vi "Max Velocity Reading.vi"() -> ()   [LabVIEW 2018]
uses:
  <vilib>/Rock Robotics/WPI/ThirdParty/Phoenix-LabVIEW/Motor Controller/Controls/CTRE_Phoenix_MotorControl_StatusFrameEnhanced.ctl
  2019_Robot_Code/Subsystems/Drive/driveShifterEnum.ctl
  <vilib>/Rock Robotics/WPI/ThirdParty/Phoenix-LabVIEW/Motor Controller/Get/CTRE_Phoenix_MotorController_GetQuadratureData.vi
panel:
  out "left Velocity (Raw Data)":i32
  out "right Velocity (Raw Data)":i32
  out "Left Max Velocity":dbl
  out "Right Max Velocity":dbl
  out "Left Max Velocity":dbl(graph)
  out "Right Max Velocity":dbl(graph)
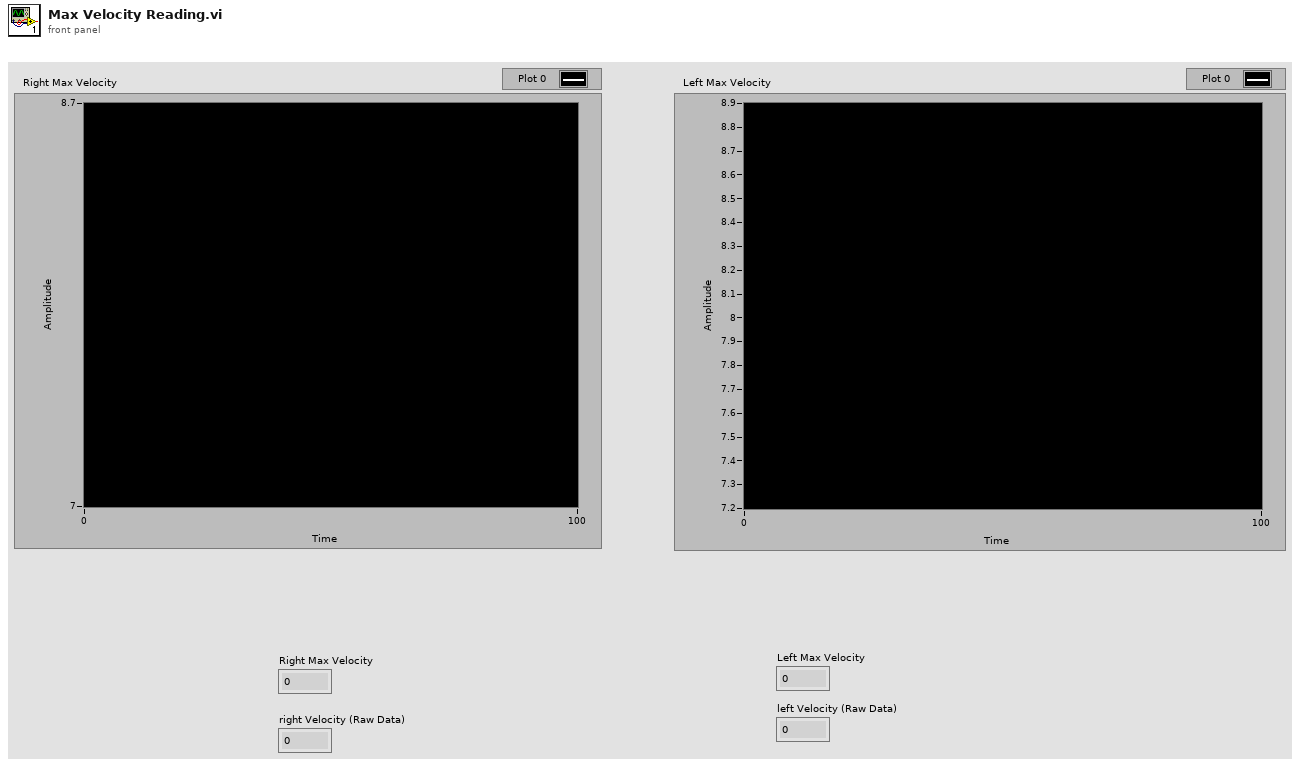
[diagram p1: front panel]
types:
  T1 = typedef "CTRE_Phoenix_MotorControl_StatusFrameEnhanced.ctl" = u16
  T2 = typedef "WPI_MotorControlDeviceRef.ctl" = cluster{"DeviceStatus":errorcluster, "Type":T3, "PWM":cluster{"PWM Channel":T4, "DeadBand":T5}, "CAN":cluster{"Device Number":u8, "SetOutput VI Ref":variant, "GetOutput VI Ref":variant, "Enable VI Ref":variant, "Disable VI Ref":variant, "Data":variant}, "Invert":bool, "DIO PWM":cluster{"PWM \"Enable\" Channel":T4, "DIOChannel":T6, "PWM Rate":dbl}}
  T3 = typedef "WPI_MotorControlType.ctl" = enum16{"PWM", "CAN", "DIO PWM"}
  T4 = typedef "FPGA_DIOPWMChannel.ctl" = enum8{"PWM 0", "PWM 1", "PWM 2", "PWM 3", "PWM 4", "PWM 5", "PWM 6", "PWM 7", "PWM 8", "PWM 9", "PWM MXP 0", "PWM MXP 1", "PWM MXP 2", "PWM MXP 3", "PWM MXP 4", "PWM MXP 5", "PWM MXP 6", "PWM MXP 7", "PWM MXP 8", "PWM MXP 9", "Invalid"}
  T5 = typedef "WPI_PWMDeadband.ctl" = cluster{"Name":string, "maxPositivePwm":i32, "minPositivePwm":i32, "centerPwm":i32, "maxNegativePwm":i32, "minNegativePwm":i32, "angularRange":u16}
  T6 = typedef "FPGA_DIOChannel.ctl" = enum8{"DIO 0", "DIO 1", "DIO 2", "DIO 3", "DIO 4", "DIO 5", "DIO 6", "DIO 7", "DIO 8", "DIO 9", "DIO MXP 0", "DIO MXP 1", "DIO MXP 2", "DIO MXP 3", "DIO MXP 4", "DIO MXP 5", "DIO MXP 6", "DIO MXP 7", "DIO MXP 8", "DIO MXP 9", "DIO MXP 10", "DIO MXP 11", "DIO MXP 12", "DIO MXP 13", "DIO MXP 14", "DIO MXP 15", "SPI Port CS1", "SPI Port CS2", "SPI Port CS3", "SPI Port MISO", "SPI Port MOSI", "Invalid"}
  T7 = enum16{"Inches -> Sensor Units", "Sensor Units -> Inches"}
  T8 = typedef "driveShifterEnum.ctl" = enum16{"Low", "High"}
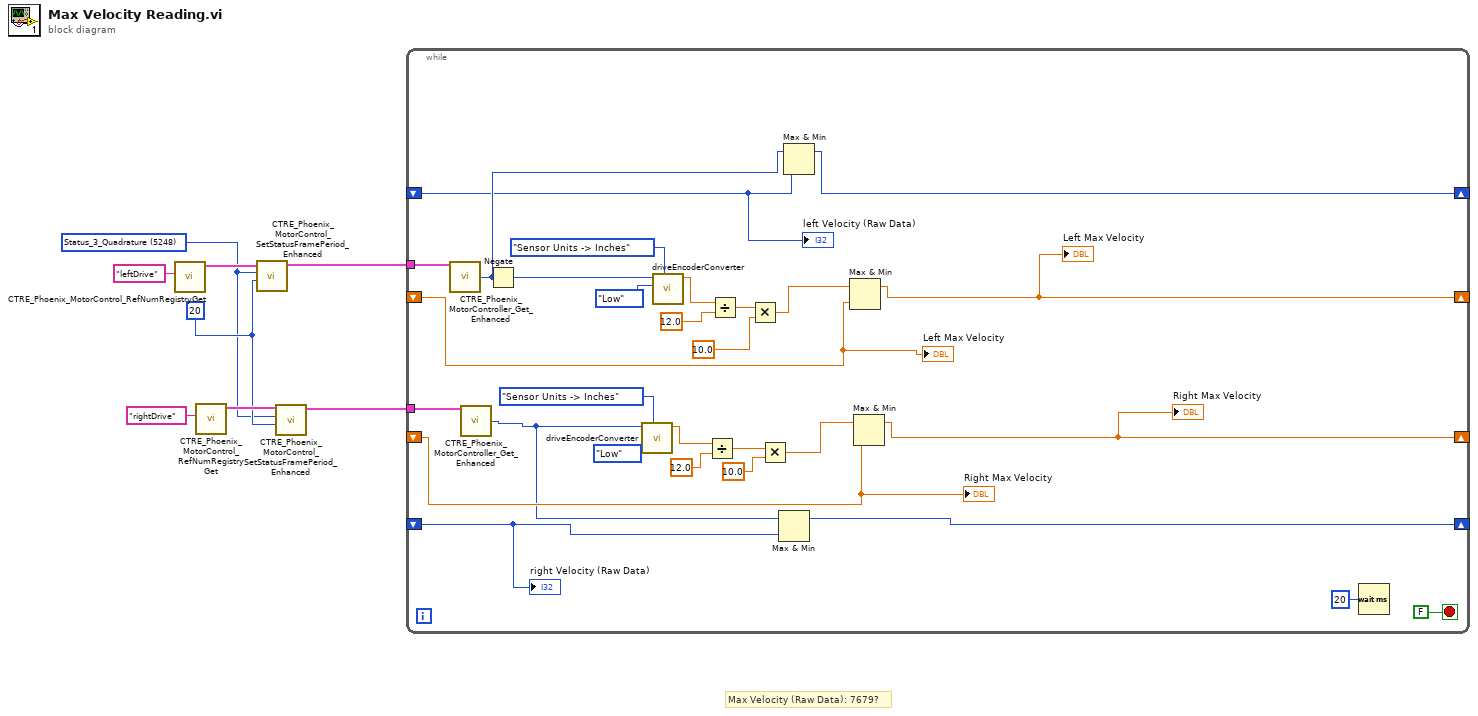
[diagram p0: block diagram]
diagram:
  w3 = T1 5248 items=["Status_1_General"=5120, "Status_2_Feedback0"=5184, "Status_3_Quadrature"=5248, "Status_4_AinTempVbat"=5312, "Status_6_Misc"=5440, "Status_7_CommStatus"=5504, "Status_8_PulseWidth"=5568, "Status_9_MotProfBuffer"=5632, "Status_10_MotionMagic"=5696, "Status_11_UartGadgeteer"=5760, "Status_12_Feedback1"=5824, "Status_13_Base_PIDF0"=5888, "Status_14_Turn_PIDF1"=5952, "Status_15_FirmwareApiStatus"=6016] ("Status Frame")
  w4 = 20 ("periodMs")
  # "Max Velocity (Raw Data): 7679?"
  n1 = call <vilib>:"CTRE_Phoenix_MotorControl_RefNumRegistryGet.vi"("refnum name"="leftDrive") -> ("PhoenixMotorControlDevRef"=w5:T2)  [unwired: 9 in, 1 out]
  n2 = call <vilib>:"CTRE_Phoenix_MotorControl_RefNumRegistryGet.vi"("refnum name"="rightDrive") -> ("PhoenixMotorControlDevRef"=w6:T2)  [unwired: 9 in, 1 out]
  n3 = call <vilib>:"CTRE_Phoenix_MotorControl_SetStatusFramePeriod_Enhanced.vi"("periodMs"=w4, "Status Frame"=w3, "PhoenixMotorControlDevRef"=w5) -> ("PhoenixMotorControlDevRef"=w2:T2)  [unwired: 7 in, 1 out]
  n4 = call <vilib>:"CTRE_Phoenix_MotorControl_SetStatusFramePeriod_Enhanced.vi"("periodMs"=w4, "Status Frame"=w3, "PhoenixMotorControlDevRef"=w6) -> ("PhoenixMotorControlDevRef"=w1:T2)  [unwired: 7 in, 1 out]
  n5 = while {
    shift-right: [w19] -> _
    shift-left: _ -> [w18]
    shift-right: [w16] -> _
    shift-left: _ -> [w15]
    tunnel: w2 -> [w35]
    tunnel: w1 -> [w34]
    shift-right: [w11] -> _
    shift-left: _ -> [w10]
    shift-right: [w13] -> _
    shift-left: _ -> [w9]
    stop <- FALSE stop-if-true
    n6 = call-poly <vilib>:"CTRE_Phoenix_MotorController_Get_Enhanced.vi"("PhoenixMotorControlDevRef"=w35) -> ("Quadrature Velocity"=w12:i32)  [unwired: 11 in, 3 out]
    n7 = call-poly <vilib>:"CTRE_Phoenix_MotorController_Get_Enhanced.vi"("PhoenixMotorControlDevRef"=w34) -> ("Quadrature Velocity"=w14:i32)  [unwired: 11 in, 3 out]
    n8 = Negate(x=w12) -> (-x=w21:i32)
    n9 = call "driveEncoderConverter.vi"("Conversion Direction"=T7."Sensor Units -> Inches", "Gear Setting"=driveShifterEnum."Low", "Input"=w14) -> ("Output"=w26:dbl)  [unwired: 8 in]
    n10 = call "driveEncoderConverter.vi"("Conversion Direction"=T7."Sensor Units -> Inches", "Gear Setting"=driveShifterEnum."Low", "Input"=w21) -> ("Output"=w31:dbl)  [unwired: 8 in]
    n11 = Divide(x=w26, y=12.0) -> (x/y=w23:dbl)
    n12 = Divide(x=w31, y=12.0) -> (x/y=w29:dbl)
    n13 = Multiply(x=w29, y=10.0) -> (x*y=w20:dbl)
    n14 = Multiply(x=w23, y=10.0) -> (x*y=w17:dbl)
    n15 = Max & Min(x=w14, y=w9) -> (max(x,y)=w13:i32)  [unwired: 1 out]
    n16 = Max & Min(x=w12, y=w10) -> (max(x,y)=w11:i32)  [unwired: 1 out]
    n17 = Max & Min(x=w20, y=w18) -> (max(x,y)=w19:dbl)  [unwired: 1 out]
    "Left Max Velocity" <- w19
    n18 = Max & Min(x=w17, y=w15) -> (max(x,y)=w16:dbl)  [unwired: 1 out]
    "Right Max Velocity" <- w16
    n19 = Wait (ms)(milliseconds to wait=u32 20) -> ()  [unwired: 1 out]
    "Left Max Velocity" <- w18
    "Right Max Velocity" <- w15
    "right Velocity (Raw Data)" <- w9
    "left Velocity (Raw Data)" <- w10
  }
